vi "UA Server Tree Test.vi"() -> ()   [LabVIEW 2017, in "Browser Core.lvlib" / "UA Server.lvclass"]
uses:
  Server Classes/UA Server/UA Server.lvclass
  <vilib>/OPCUA/controls/NodeId.ctl
  Server Classes/UA Server/UA Server.lvclass/UA Server.ctl
  C:/Users/MattJ/Desktop/GitHubSCM/UA-Server-Browser/source/Browser Core/Server Classes/Base Tree/Base Tree.lvclass
  <vilib>/OPCUA/NI OPC UA Utility.lvlib
  <vilib>/OPCUA/NI OPC UA Client.lvlib
  Server Classes/Base Tree/Base Tree.lvclass
panel:
  in  "Tree":string(tree)
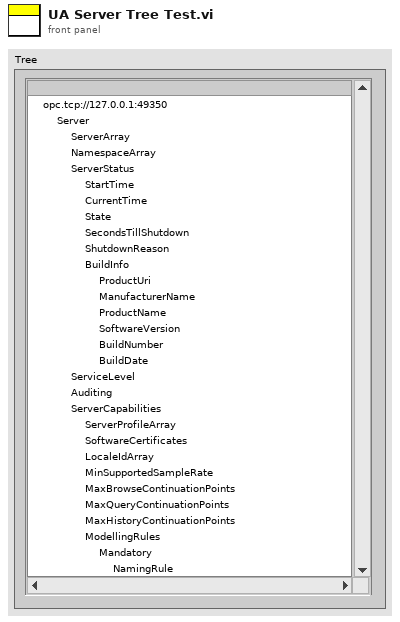
[diagram p1: front panel]
types:
  T1 = typedef "NodeId.ctl" = string
  T2 = cluster{"message mode":enum16{"None", "Sign", "Sign and Encrypt"}, "security":enum16{"Basic256", "Basic128Rsa15"}}
  T3 = typedef "OPC UA Client Refnum.ctl" = refnum<k21>
  T4 = typedef "Node Class.ctl" = u32
  T5 = cluster{"reference type":u32, "node ID":T1, "browse name":string, "node class":T4, "node type":u32}[]
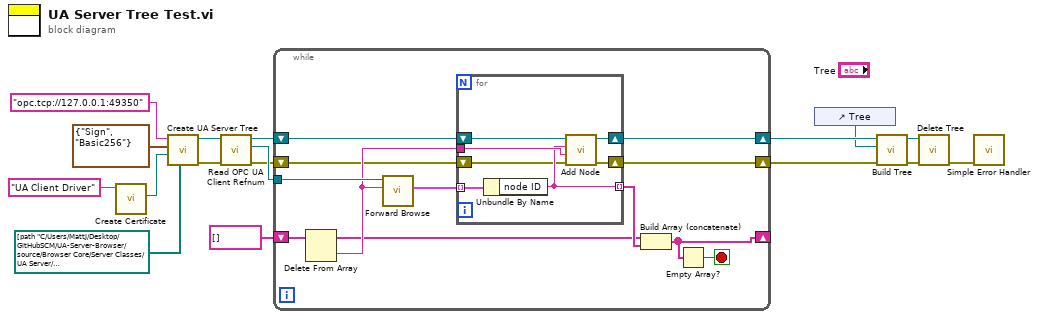
[diagram p0: block diagram]
diagram:
  n1 = call <vilib>:"Create Certificate.vi"("certificate name in"="UA Client Driver") -> ("certificate path"=w14:path)  [unwired: 7 in, 3 out]
  n2 = call "Create UA Server Tree.vi"("Trusted Server Certificates"=path[] [path "C:/Users/MattJ/Desktop/GitHubSCM/UA-Server-Browser/source/Browser Core/Server Classes/UA Server/d418c6502bb465e37e4056aec0cd6473014210cc.der"], "Client Certificate File"=w14, "Security Policy"=T2 {"message mode"=enum."Sign", "security"=enum."Basic256"} ("security policy"), "Server Endpoint URL"="opc.tcp://127.0.0.1:49350" ("server endpoint URL")) -> ("Error Out"=w12:errorcluster, "UA Server Tree"=w11:refnum<class "UA Server.lvclass">)  [unwired: 6 in]
  n3 = call "Read OPC UA Client Refnum.vi"("error in (no error)"=w12, "UA Server in"=w11) -> ("error out"=w4:errorcluster, "OPC UA client refnum"=w6:T3, "UA Server out"=w10:refnum<class "UA Server.lvclass">)  [unwired: 7 in]
  n4 = while {
    shift-right: [w22] -> w9
    shift-left: w10 -> [w28]
    shift-right: [w24] -> _
    shift-left: T1[] [] -> [w21]
    tunnel: w6 -> [w29]
    shift-right: [w18] -> w3
    shift-left: w4 -> [w19]
    stop <- w23 stop-if-true
    n5 = Delete From Array(array=w21) -> (deleted portion=w26:T1, array with subset deleted=w20:T1[])  [unwired: 2 in]
    n6 = call <vilib>:"Forward Browse.vi"("node ID"=w26, "OPC UA client refnum in"=w29) -> ("browse result"=w27:T5)  [unwired: 6 in, 3 out]
    n7 = for {
      tunnel: w27 -> [w35] mode=indexing
      tunnel: w26 -> [w34]
      tunnel: [w33] -> w25 mode=indexing
      shift-right: [w32] -> w22
      shift-left: w28 -> [w36]
      shift-right: [w30] -> w18
      shift-left: w19 -> [w31]
      n8 = Unbundle By Name(w35) -> ("node ID"=w33:T1)
      n9 = call-dynamic "Add Node.vi"("error in (no error)"=w31, "Parent"=w34, "UID"=w33, "Base Tree in"=w36) -> ("error out"=w30:errorcluster, "Base Tree out"=w32:refnum<class "UA Server.lvclass">)  [unwired: 6 in]
    }
    n10 = Build Array (concatenate)(w20, w25) -> (w24:T1[])
    n11 = Empty Array?(array=w24) -> (empty?=w23:bool)
  }
  n12 = control-ref of="Tree"() -> (w8:refnum<vi>)
  n13 = call "Build Tree.vi"("error in (no error)"=w3, "Tree Reference"=w8, "Base Tree in"=w9) -> ("error out"=w2:errorcluster, "Base Tree out"=w7:refnum<class "UA Server.lvclass">)  [unwired: 7 in]
  n14 = call-dynamic "Delete Tree.vi"("error in (no error)"=w2, "UA Server in"=w7) -> ("error out"=w1:errorcluster)  [unwired: 9 in]
  n15 = call <vilib>:"Simple Error Handler.vi"("error in (no error)"=w1) -> ()  [unwired: 4 in, 5 out]
